vi "Main.vi"(11 "Actor Script Strategy in":refnum<class "Actor Script Strategy.lvclass">) -> ()   [LabVIEW 2021, in "_Create From Template.lvlib" / "Script Strategy.lvlib" / "Actor Script Strategy.lvclass"]
uses:
  Actor Script Strategy.lvclass
  Actor Script Strategy.lvclass/Actor Script Strategy.ctl
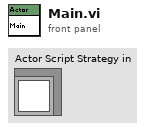
[diagram p1: front panel]
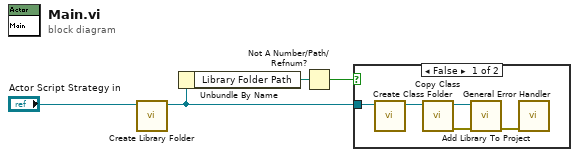
[diagram p0: block diagram]
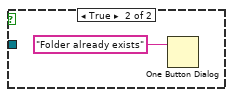
[diagram p2: hidden frame]
diagram:
  n1 = call-dynamic "Create Library Folder.vi"("Actor Script Strategy in"="Actor Script Strategy in") -> ("Actor Script Strategy out"=w3:refnum<class "Actor Script Strategy.lvclass">)  [unwired: 10 in]
  n2 = Unbundle By Name(w3) -> ("Library Folder Path"=w2:path)
  n3 = Not A Number/Path/Refnum?(number/path/refnum=w2) -> (NaN/Path/Refnum?=w1:bool)
  n4 = case shown="False" w1 {
    tunnel: w3 -> [w6 _]
    frame False {
      n5 = call-dynamic "Create Class Folder.vi"("Actor Script Strategy in"=w6) -> ("Actor Script Strategy out"=w5:refnum<class "Actor Script Strategy.lvclass">)  [unwired: 10 in]
      n6 = call-dynamic "Copy Class.vi"("Actor Script Strategy in"=w5) -> ("error out"=w8:errorcluster, "Actor Script Strategy out"=w7:refnum<class "Actor Script Strategy.lvclass">)  [unwired: 9 in]
      n7 = call-dynamic "Add Library To Project.vi"("error in"=w8, "Actor Script Strategy in"=w7) -> ("error out"=w9:errorcluster)  [unwired: 9 in]
      n8 = call <vilib>:"General Error Handler.vi"("error in (no error)"=w9) -> ()  [unwired: 10 in, 5 out]
    }
    frame True {
      n9 = One Button Dialog(message="Folder already exists") -> ()  [unwired: 1 in, 1 out]
    }
  }
